vi "旁路启动参数.vi"() -> ()   [LabVIEW 2016, in "质控单元V4.lvlib"]
uses:
  <vilib>/Utility/config.llb/NI_LVConfig.lvlib
panel:
  in  "启用参数":T1
  in  "关闭":bool
  in  "保存":bool
  out "启动参数":string
  # "请选择要启动的参数"
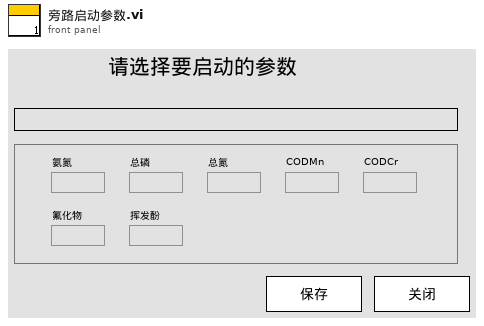
[diagram p1: front panel]
types:
  T1 = cluster{"氨氮":bool, "总磷":bool, "总氮":bool, "CODMn":bool, "CODCr":bool, "氟化物":bool, "挥发酚":bool}
  T2 = typedef "NI_LVConfig.lvlib/Config Data RefNum.ctl" = refnum<k1>
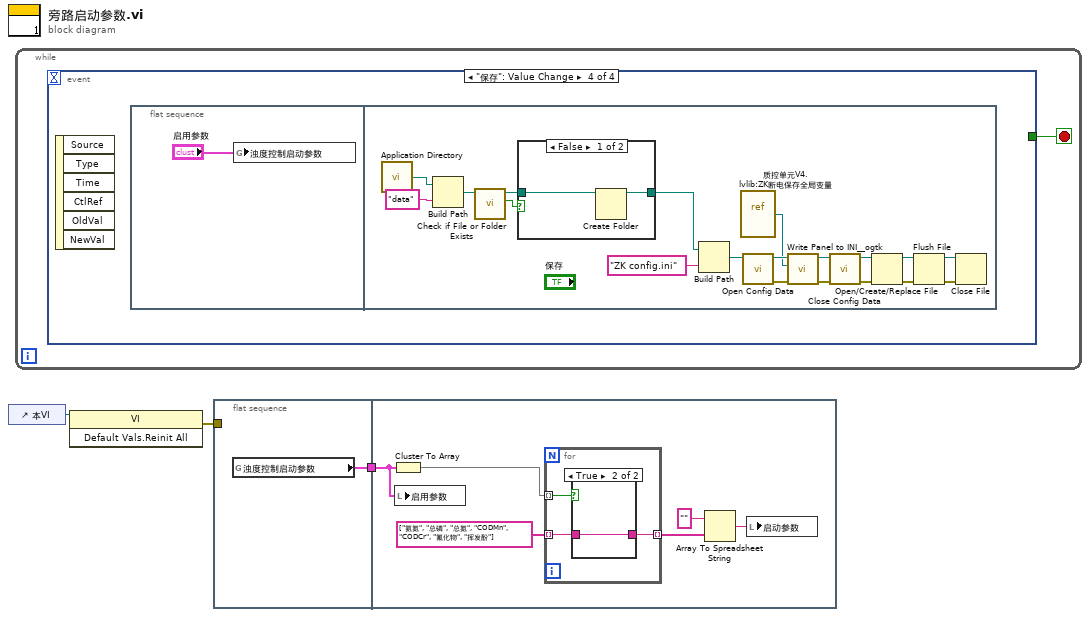
[diagram p0: block diagram]
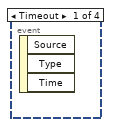
[diagram p3: hidden frame]
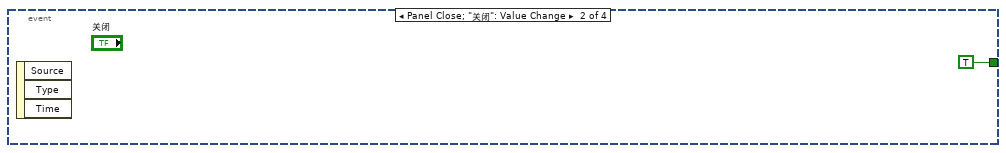
[diagram p4: hidden frame]
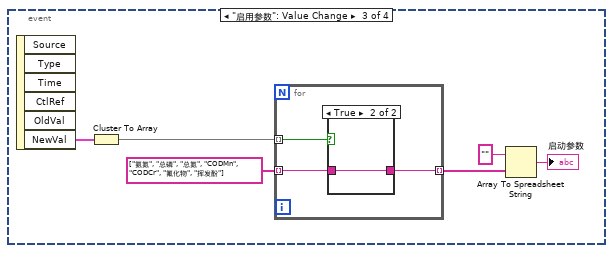
[diagram p5: hidden frame]
diagram:
  n1 = control-ref of="本VI"() -> (w3:refnum<vi>)
  n2 = while {
    stop <- w4 stop-if-true
    n3 = event shown="[3] \"保存\": Value Change" {
      selector: _ -> [_ _ _ _]
      dyn-events: _ -> [_ _ _ _]
      timeout: _ -> [_ _ _ _]
      tunnel: [_ TRUE _ _] -> w4
      event Timeout {
        n4 = event-data() -> ()  [unwired: 1 in, 3 out]
      }
      event Panel Close; "关闭": Value Change {
        n5 = event-data() -> ()  [unwired: 1 in, 3 out]
      }
      event "启用参数": Value Change {
        n6 = event-data() -> ("NewVal"=w6:T1)  [unwired: 1 in, 5 out]
        n7 = Cluster To Array(cluster=w6) -> (array=w11:bool[])
        n8 = for {
          tunnel: w11 -> [w14] mode=indexing
          tunnel: string[] ["氨氮", "总磷", "总氮", "CODMn", "CODCr", "氟化物", "挥发酚"] -> [w13] mode=indexing
          tunnel: [w12] -> w8 mode=indexing
          n9 = case shown="True" w14 {
            tunnel: w13 -> [_ w15]
            tunnel: [_ w15] -> w12
            frame False {
            }
            frame True {
            }
          }
        }
        n10 = Array To Spreadsheet String(array=w8, 3:"" ("格式字符串")) -> (spreadsheet string=→"启动参数":string)  [unwired: 1 in]
      }
      event "保存": Value Change {
        n11 = event-data() -> ()  [unwired: 1 in, 6 out]
        n12 = flat-sequence {
          frame #0 {
            n13 = global write "ZK断电保存全局变量.vi" "浊度控制启动参数"("启用参数") -> ()
          }
          frame #1 {
            n14 = call <vilib>:"Application Directory.vi"() -> ("Application Directory"=w18:path)
            n15 = Build Path(base path=w18, name or relative path="data" ("名称或相对路径")) -> (appended path=w20:path)
            n16 = call <vilib>:"Check if File or Folder Exists.vi"("path"=w20) -> ("file or folder exists?"=w21:bool, "dup path"=w22:path)  [unwired: 8 in, 1 out]
            n17 = case shown="False" w21 {
              tunnel: w22 -> [w37 w38]
              tunnel: [w36 w38] -> w23
              frame False {
                n18 = Create Folder(path (use dialog)=w37) -> (created path=w36:path)  [unwired: 2 in, 2 out]
              }
              frame True {
              }
            }
            n19 = Build Path(base path=w23, name or relative path="ZK config.ini" ("名称或相对路径")) -> (appended path=w17:path)
            n20 = vi-ref "质控单元V4.lvlib:ZK断电保存全局变量.vi"() -> (w25:refnum<vi>)
            n21 = call <vilib>:"Open Config Data.vi"("configuration file path"=w17) -> ("error out"=w28:errorcluster, "refnum"=w26:T2)  [unwired: 8 in, 1 out]
            n22 = call <userlib>:"Write Panel to INI__ogtk.vi"("error in (no error)"=w28, "VI ref"=w25, "refnum"=w26) -> ("error out"=w29:errorcluster, "refnum out"=w27:T2)  [unwired: 7 in]
            n23 = call <vilib>:"Close Config Data.vi"("error in (no error)"=w29, "refnum"=w27) -> ("error out"=w34:errorcluster, "file path"=w35:path)  [unwired: 8 in]
            n24 = Open/Create/Replace File(file path (use dialog)=w35, error in=w34) -> (refnum out=w31:refnum<file>, error out=w30:errorcluster)  [unwired: 4 in, 1 out]
            n25 = Flush File(refnum=w31, error in=w30) -> (refnum out=w32:refnum<file>, error out=w33:errorcluster)
            n26 = Close File(refnum=w32, error in=w33) -> ()  [unwired: 2 out]
          }
        }
      }
    }
  }
  n27 = invoke class="VI" method="Default Vals.Reinit All"(reference=w3) -> (error out=w2:errorcluster)  [unwired: 2 in, 2 out]
  n28 = flat-sequence {
    tunnel: w2 -> [_]
    tunnel: [w39] -> w1
    tunnel: w1 -> [w40]
    frame #0 {
      n29 = global read "ZK断电保存全局变量.vi" "浊度控制启动参数"() -> (w39:T1)
    }
    frame #1 {
      n30 = Cluster To Array(cluster=w40) -> (array=w43:bool[])
      n31 = local write "启用参数"(w40) -> ()
      n32 = for {
        tunnel: w43 -> [w48] mode=indexing
        tunnel: string[] ["氨氮", "总磷", "总氮", "CODMn", "CODCr", "氟化物", "挥发酚"] -> [w47] mode=indexing
        tunnel: [w46] -> w41 mode=indexing
        n33 = case shown="True" w48 {
          tunnel: w47 -> [_ w49]
          tunnel: [_ w49] -> w46
          frame False {
          }
          frame True {
          }
        }
      }
      n34 = Array To Spreadsheet String(array=w41, 3:"" ("格式字符串")) -> (spreadsheet string=w44:string)  [unwired: 1 in]
      n35 = local write "启动参数"(w44) -> ()
    }
  }
